vi "自由间隙.vi"(0 "曲线引用":refnum<vi>, 1 "自由间隙判定条件":cluster{"下限":dbl, "上限":dbl}, 3 "错误输入":errorcluster) -> (7 "曲线引用输出":refnum<vi>, 8 "OK？":bool, 10 "错误输出":errorcluster)   [LabVIEW 2017]
uses:
  Global_Variable/Global.vi
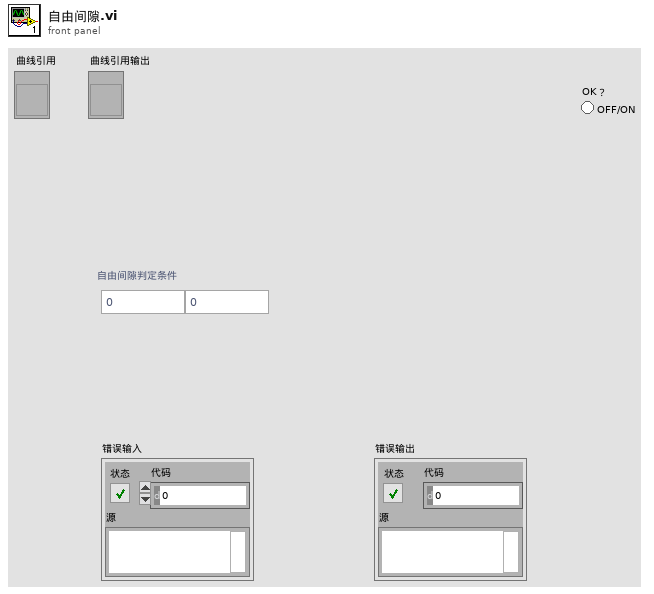
[diagram p1: front panel]
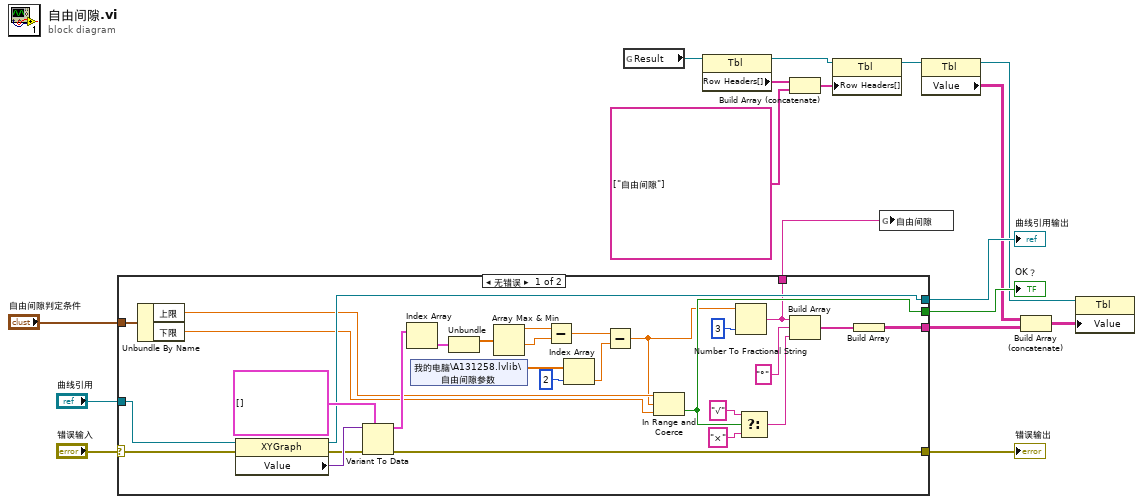
[diagram p0: block diagram]
diagram:
  n1 = case shown="无错误" "错误输入" {
    selector: "错误输入" -> [w44 w48]
    tunnel: [w41 w48] -> w16
    tunnel: "曲线引用" -> [w40 w47]
    tunnel: [w43 w47] -> w14
    tunnel: [w27 _] -> w13
    tunnel: "自由间隙判定条件" -> [w30 _]
    tunnel: [w31 _] -> w9
    tunnel: [w18 _] -> w1
    frame No Error {
      n2 = Unbundle By Name(w30) -> ("上限"=w29:dbl, "下限"=w28:dbl)
      n3 = property class="XYGraph"(reference=w40, error in=w44) -> (reference out=w43:refnum<vi>, error out=w42:errorcluster, "Value"=w46:variant)
      n4 = Variant To Data(error in=w42, type=cluster{dbl[], dbl[]}[] [], Variant=w46) -> (data=w34:cluster{dbl[], dbl[]}[], error out=w41:errorcluster)
      n5 = Index Array(array=w34) -> (element=w33:cluster{dbl[], dbl[]})  [unwired: 1 in]
      n6 = shared-variable "我的电脑\\A131258.lvlib\\自由间隙参数"() -> (w22:sgl[])  [unwired: 1 in, 1 out]
      n7 = Unbundle(w33) -> (w26:dbl[])  [unwired: 1 out]
      n8 = Array Max & Min(array=w26) -> (max value=w25:dbl, min value=w24:dbl)  [unwired: 2 out]
      n9 = Subtract(x=w25, y=w24) -> (x-y=w23:dbl)
      n10 = Index Array(array=w22, index=2 ("索引")) -> (element=w20:sgl)
      n11 = Subtract(x=w23, y=w20) -> (x-y=w19:dbl)
      n12 = In Range and Coerce(upper limit=w29, x=w19, lower limit=w28) -> (In Range?=w27:bool)  [unwired: 1 out]
      n13 = Number To Fractional String(number=w19, precision (6)=i16 3 ("精度(6)")) -> (F-format string=w18:string)  [unwired: 2 in]
      n14 = Select(t="√" ("元素"), s=w27, f="×" ("元素")) -> (s? t:f=w35:string)
      n15 = Build Array(w18, "°" ("元素"), w35) -> (w32:string[])
      n16 = Build Array(w32) -> (w31:string[][])
    }
    frame Error {
    }
  }
  "错误输出" <- w16
  "曲线引用输出" <- w14
  "OK？" <- w13
  n17 = global read "Global.vi" "Result"() -> (w8:refnum<vi>)
  n18 = property class="Tbl"(reference=w8) -> (reference out=w7:refnum<vi>, "Row Headers[]"=w5:string[])  [unwired: 1 in, 1 out]
  n19 = Build Array (concatenate)(w5, string[] ["自由间隙"] ("列首字符串[]")) -> (w3:string[])
  n20 = property class="Tbl"(reference=w7, "Row Headers[]"=w3) -> (reference out=w6:refnum<vi>)  [unwired: 1 in, 1 out]
  n21 = global write "检测结果.vi" "自由间隙"(w1) -> ()
  n22 = property class="Tbl"(reference=w6) -> (reference out=w12:refnum<vi>, "Value"=w11:string[][])  [unwired: 1 in, 1 out]
  n23 = Build Array (concatenate)(w11, w9) -> (w10:string[][])
  n24 = property class="Tbl"(reference=w12, "Value"=w10) -> ()  [unwired: 1 in, 2 out]
